vi "Display IMAQ at Monitor with NI-VISION.vi"() -> ()   [LabVIEW 2017]
uses:
  IMAQCV/IMAQCV.lvlib
  IMAQCV/LVOpenCV.lvlib
panel:
  in  "Image Delay ms":u32=5000
  in  "Image File path":path=path "c:/vision/Metal1.jpg"
  out "Image Log path":path=path "c:/vision/Result.jpg"
  out "Image Out 3":T1(plugin-control)
  out "Number of Particles":i32
  out "error out":errorcluster
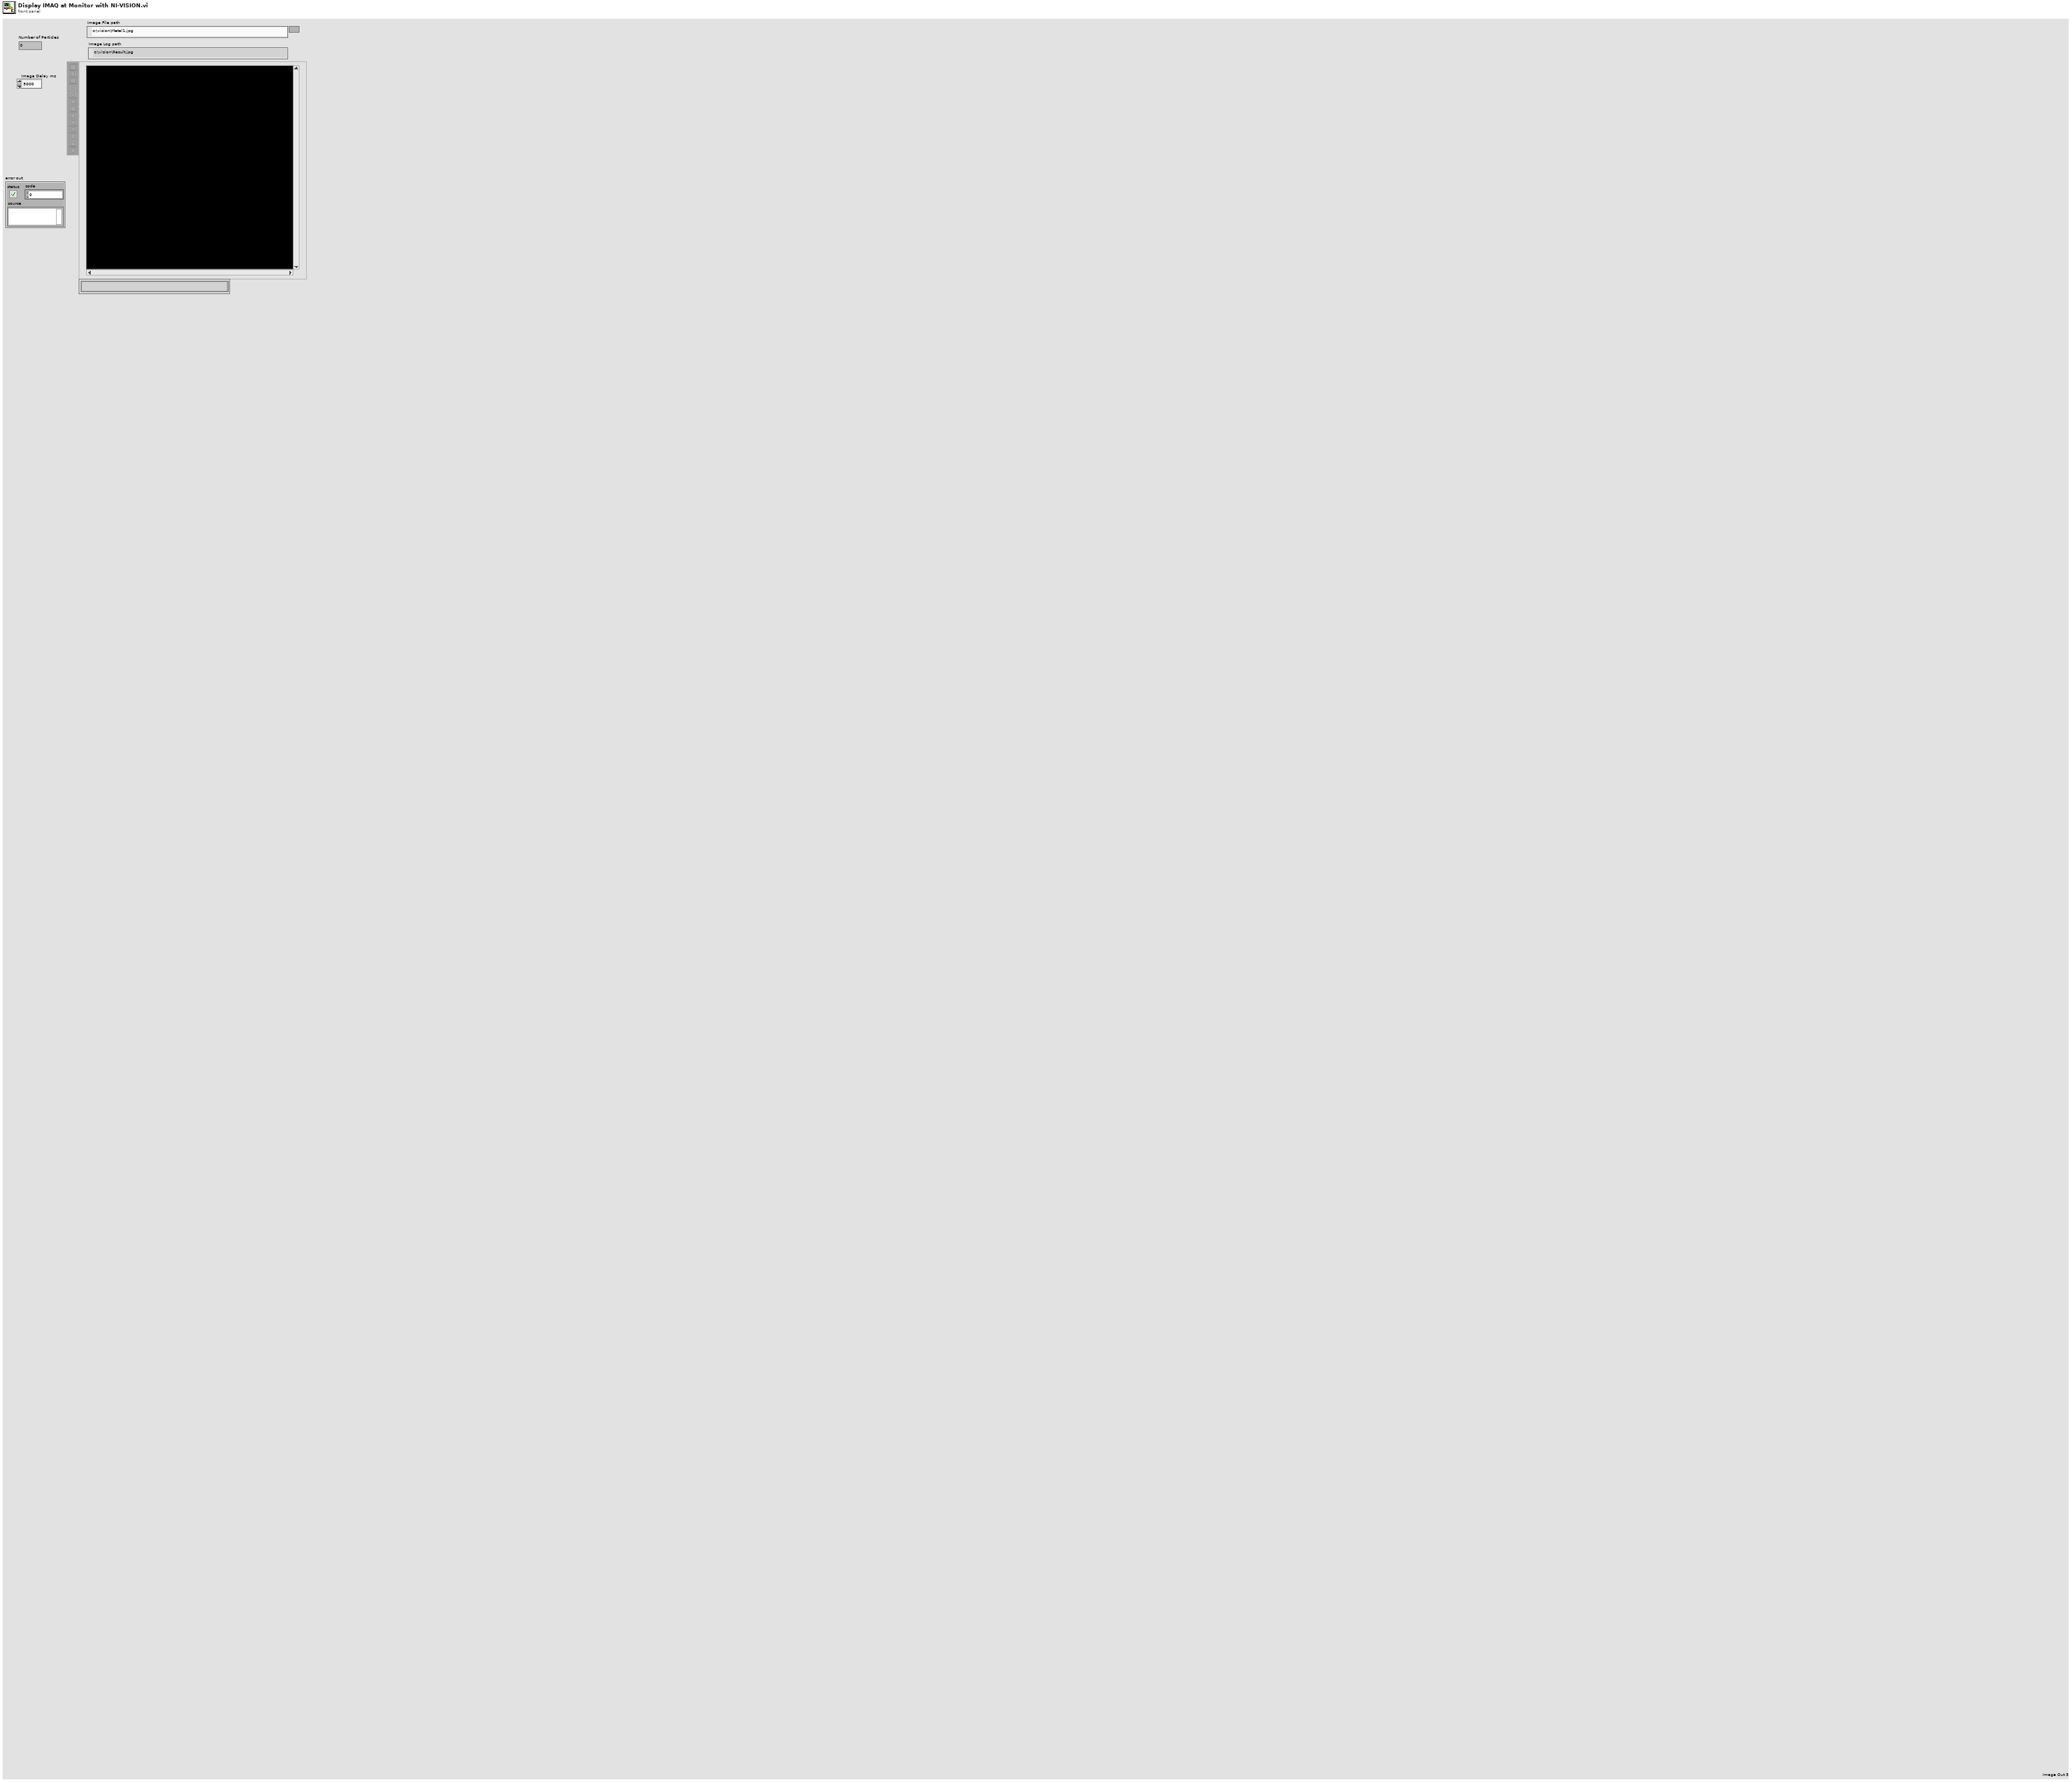
[diagram p1: front panel]
types:
  T1 = typedef "IMAQ Image.ctl" = refnum<image>
  T2 = typedef "Image Type" = u32
  T3 = typedef "IMAQCV.lvlib/IMAQCV Image.ctl" = refnum<vi>
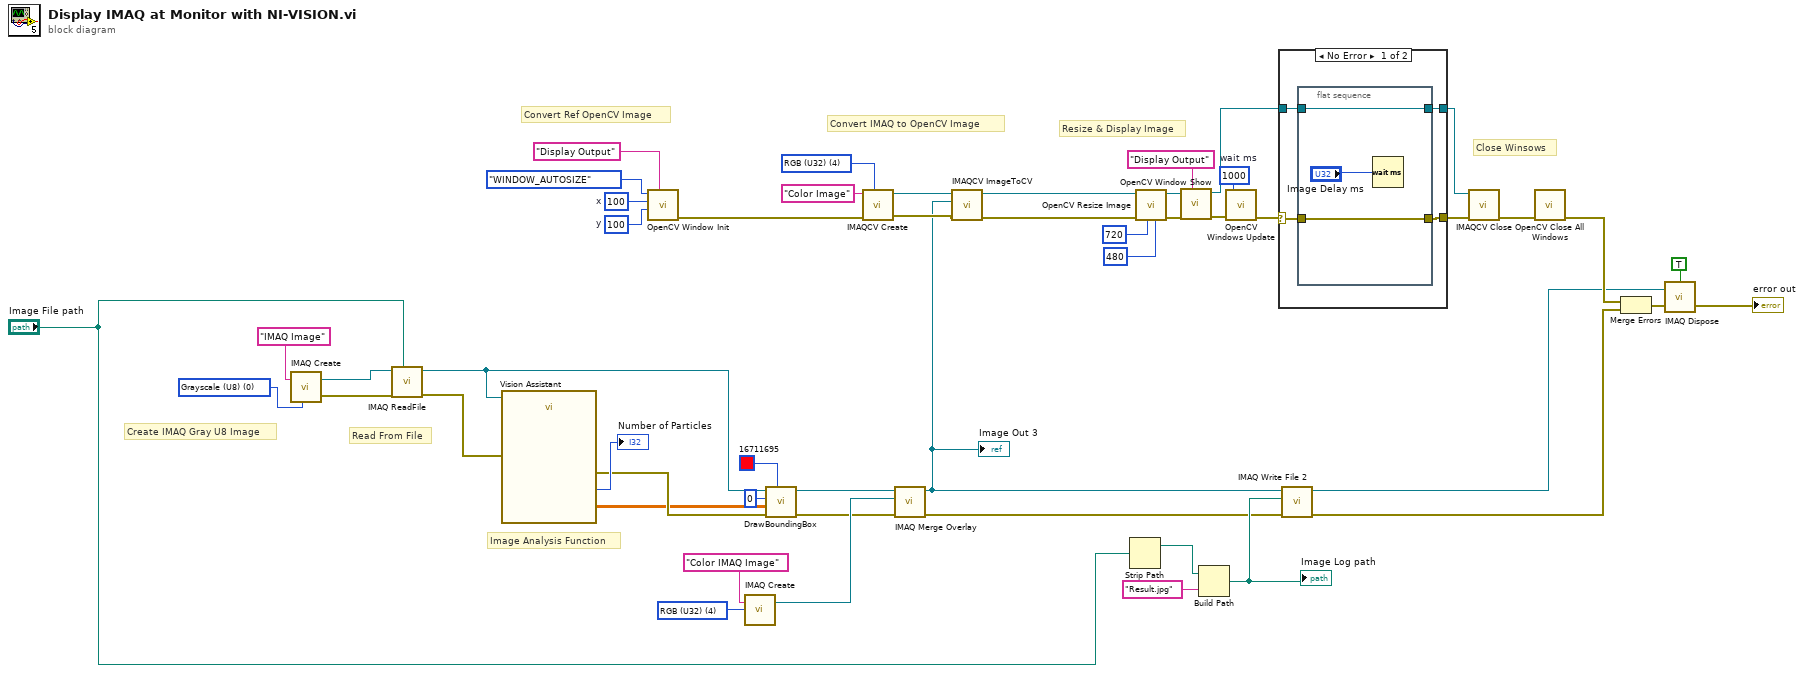
[diagram p0: block diagram]
diagram:
  w20 = 1000  # wait ms
  w27 = u32 100  # y
  w28 = u32 100  # x
  w31 = u32 4 items=["Grayscale (U8)", "Grayscale (I16)", "Grayscale (SGL)", "Complex (CSG)", "RGB (U32)", "HSL (U32)", "RGB (U64)", "Grayscale (U16)"] ("Image Type")
  w40 = T2 4 items=["Grayscale (U8)", "Grayscale (I16)", "Grayscale (SGL)", "Complex (CSG)", "RGB (U32)", "HSL (U32)", "RGB (U64)", "Grayscale (U16)"] ("Image Type")
  w48 = T2 0 items=["Grayscale (U8)", "Grayscale (I16)", "Grayscale (SGL)", "Complex (CSG)", "RGB (U32)", "HSL (U32)", "RGB (U64)", "Grayscale (U16)"] ("Image Type")
  # "Close Winsows"
  # "Resize & Display Image"
  # "Convert Ref OpenCV Image"
  # "Convert IMAQ to OpenCV Image"
  # "Image Analysis Function"
  # "Read From File"
  # "Create IMAQ Gray U8 Image"
  n1 = call "IMAQ Create"("Image Name"="IMAQ Image", "Image Type"=w48) -> ("New Image"=w50:T1, "error out"=w49:errorcluster)  [unwired: 2 in, 1 out]
  n2 = call "IMAQ ReadFile"("File Path"="Image File path", "error in (no error)"=w49, "Image"=w50) -> ("error out"=w47:errorcluster, "Image Out"=w2:T1)  [unwired: 2 in, 5 out]
  n3 = call "Vision Assistant"("Image In"=w2, "error in"=w47) -> ("Number of Particles (Particle Analysis 1)"=→"Number of Particles":i32, "Particle Measurements (Pixels) (Particle Analysis 1)"=w44:dbl[][], "error out"=w45:errorcluster)  [unwired: 22 in, 1 out]
  n4 = call "OpenCV Window Init.vi"("window name"="Display Output", "y"=w27, "x"=w28, "mode"=enum8{"WINDOW_AUTOSIZE", "WINDOW_FULLSCREEN"}."WINDOW_AUTOSIZE") -> ("error out"=w11:errorcluster)  [unwired: 7 in]
  n5 = call "IMAQ Create"("Image Name"="Color IMAQ Image", "Image Type"=w40) -> ("New Image"=w38:T1)  [unwired: 2 in, 2 out]
  n6 = call "DrawBoundingBox.vi"("Color"=u32 16711695, "error in (no error)"=w45, "Particle Measurements"=w44, "index of Bounding Rect Left"=0, "Image"=w2) -> ("error out"=w5:errorcluster, "Image 2"=w39:T1)  [unwired: 5 in]
  n7 = call "IMAQCV Create.vi"("Image Type"=w31, "error in (no error)"=w11, "Image Name"="Color Image") -> ("error out"=w14:errorcluster, "Image Out"=w32:T3)  [unwired: 7 in]
  n8 = call "IMAQ Merge Overlay"("error in (no error)"=w5, "Image Dst"=w38, "Image Src"=w39) -> ("error out"=w4:errorcluster, "Image Dst Out"=w1:T1)  [unwired: 7 in]
  "Image Out 3" <- w1
  n9 = call "IMAQCV ImageToCV.vi"("error in (no error)"=w14, "Variant In"=w1, "CV in"=w32) -> ("error out"=w10:errorcluster, "CV out"=w19:T3)  [unwired: 7 in]
  n10 = Strip Path(path="Image File path") -> (stripped path=w36:path)  [unwired: 1 out]
  n11 = call "OpenCV Resize Image.vi"("height"=u32 480, "width"=u32 720, "error in (no error)"=w10, "image in"=w19) -> ("error out"=w23:errorcluster, "image out"=w24:T3)  [unwired: 6 in]
  n12 = call "OpenCV Window Show.vi"("window name"="Display Output", "error in (no error)"=w23, "image in"=w24) -> ("error out"=w25:errorcluster, "image out"=w17:T3)  [unwired: 7 in]
  n13 = Build Path(base path=w36, name or relative path="Result.jpg") -> (appended path=w34:path)
  "Image Log path" <- w34
  n14 = call "OpenCV Windows Update.vi"("error in (no error)"=w25, "wait ms"=w20) -> ("error out"=w13:errorcluster)  [unwired: 8 in, 1 out]
  n15 = case shown="No Error" w13 {
    selector: w13 -> [w52 w60]
    tunnel: [w55 w60] -> w18
    tunnel: w17 -> [w54 w59]
    tunnel: [w53 w59] -> w16
    frame No Error {
      n16 = flat-sequence {
        tunnel: [w58] -> w55
        tunnel: w52 -> [w58]
        tunnel: [w57] -> w53
        tunnel: w54 -> [w57]
        frame #0 {
          n17 = Wait (ms)(milliseconds to wait="Image Delay ms") -> ()  [unwired: 1 out]
        }
      }
    }
    frame Error {
    }
  }
  n18 = call-poly "IMAQ Write File 2"("error in (no error)"=w4, "File Path"=w34, "Image"=w1) -> ("error out"=w3:errorcluster, "Image Out (duplicate)"=w7:T1)  [unwired: 7 in]
  n19 = call "IMAQCV Close.vi"("error in (no error)"=w18, "Image"=w16) -> ("error out"=w15:errorcluster)  [unwired: 9 in]
  n20 = call "OpenCV Close All Windows.vi"("error in (no error)"=w15) -> ("error out"=w8:errorcluster)  [unwired: 10 in]
  n21 = Merge Errors(w8, w3) -> (w9:errorcluster)
  n22 = call "IMAQ Dispose"("All Images? (No)"=TRUE, "Image"=w7, "error in (no error)"=w9) -> ("error out"=→"error out":errorcluster)  [unwired: 3 in]
